vi "start cases.vi"() -> ()   [LabVIEW 2015]
panel:
  out "right pwm out":dbl
  out "left pwm out":dbl
  in  "Tab Control":T1(tab)
  in  "right 0":dbl
  in  "left 0":dbl
  in  "left 1":dbl
  in  "right 1":dbl
  in  "left 2 straight":dbl
  in  "right 2 straight":dbl
  in  "right 2 arc":dbl
  in  "left 2 arc":dbl
  in  "left 3 arc 1":dbl
  in  "right 3 arc 1":dbl
  in  "left 3 arc 2":dbl
  in  "right 3 arc 2":dbl
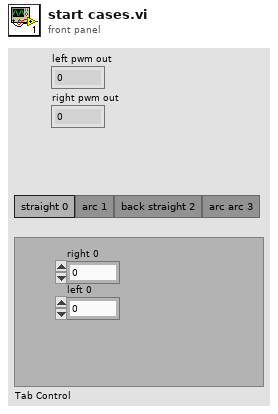
[diagram p1: front panel]
types:
  T1 = enum32{"straight 0", "arc 1", "back straight 2", "arc arc 3"}
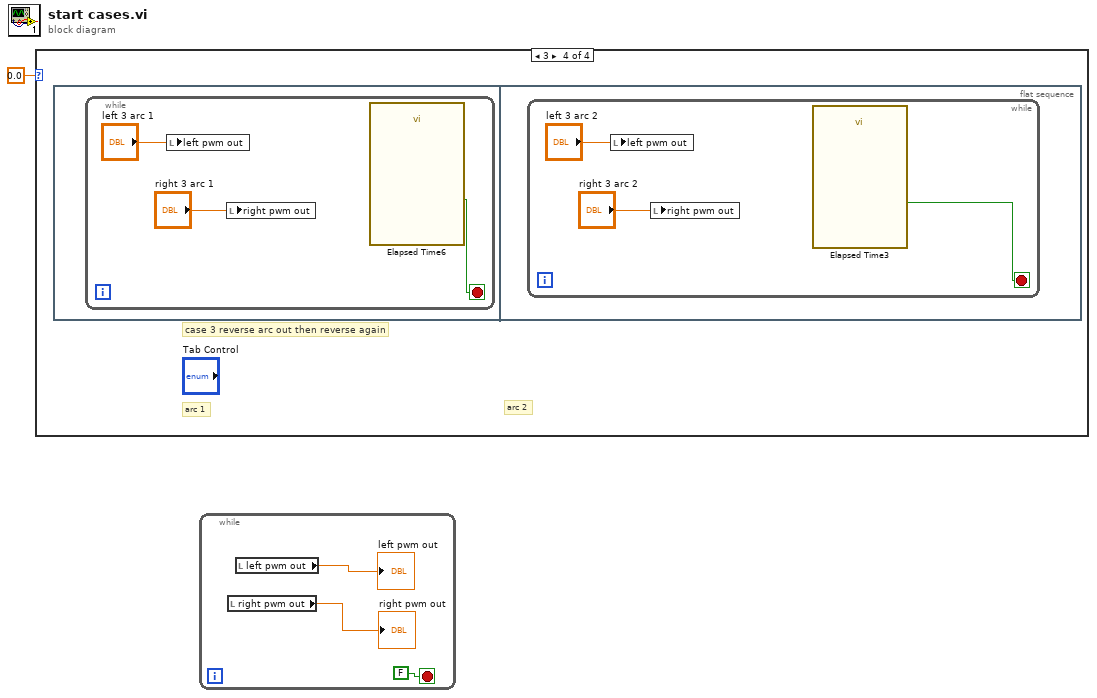
[diagram p0: block diagram]
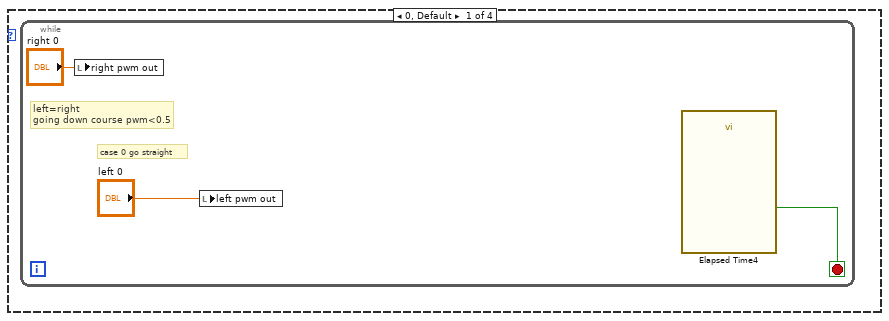
[diagram p2: hidden frame]
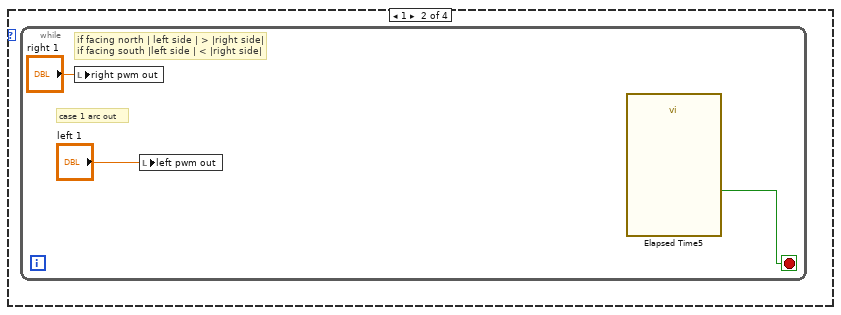
[diagram p3: hidden frame]
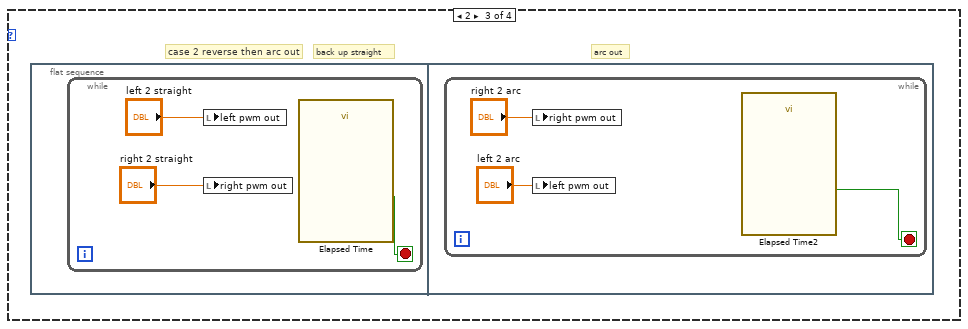
[diagram p4: hidden frame]
diagram:
  n1 = case shown="3" 0.0 {
    frame 0, Default {
      n2 = while {
        stop <- w2 stop-if-true
        # "left=right\ngoing down course pwm<0.5"
        # "case 0 go straight"
        n3 = local write "right pwm out"("right 0") -> ()
        n4 = local write "left pwm out"("left 0") -> ()
        n5 = call "Elapsed Time4"() -> ("Time has Elapsed"=w2:bool)  [unwired: 12 in, 7 out]
      }
    }
    frame 1 {
      n6 = while {
        stop <- w5 stop-if-true
        # "if facing north | left side | > |right side|\nif facing south |left side | < |right side|"
        # "case 1 arc out"
        n7 = local write "right pwm out"("right 1") -> ()
        n8 = local write "left pwm out"("left 1") -> ()
        n9 = call "Elapsed Time5"() -> ("Time has Elapsed"=w5:bool)  [unwired: 12 in, 7 out]
      }
    }
    frame 2 {
      # "arc out"
      # "back up straight"
      # "case 2 reverse then arc out"
      n10 = flat-sequence {
        frame #0 {
          n11 = while {
            stop <- w8 stop-if-true
            n12 = local write "left pwm out"("left 2 straight") -> ()
            n13 = local write "right pwm out"("right 2 straight") -> ()
            n14 = call "Elapsed Time"() -> ("Time has Elapsed"=w8:bool)  [unwired: 12 in, 7 out]
          }
        }
        frame #1 {
          n15 = while {
            stop <- w11 stop-if-true
            n16 = local write "right pwm out"("right 2 arc") -> ()
            n17 = local write "left pwm out"("left 2 arc") -> ()
            n18 = call "Elapsed Time2"() -> ("Time has Elapsed"=w11:bool)  [unwired: 12 in, 7 out]
          }
        }
      }
    }
    frame 3 {
      # "arc 2"
      # "arc 1"
      # "case 3 reverse arc out then reverse again"
      n19 = flat-sequence {
        frame #0 {
          n20 = while {
            stop <- w14 stop-if-true
            n21 = local write "left pwm out"("left 3 arc 1") -> ()
            n22 = local write "right pwm out"("right 3 arc 1") -> ()
            n23 = call "Elapsed Time6"() -> ("Time has Elapsed"=w14:bool)  [unwired: 12 in, 7 out]
          }
        }
        frame #1 {
          n24 = while {
            stop <- w17 stop-if-true
            n25 = local write "left pwm out"("left 3 arc 2") -> ()
            n26 = local write "right pwm out"("right 3 arc 2") -> ()
            n27 = call "Elapsed Time3"() -> ("Time has Elapsed"=w17:bool)  [unwired: 12 in, 7 out]
          }
        }
      }
    }
  }
  n28 = while {
    stop <- FALSE stop-if-true
    n29 = local read "right pwm out"() -> (→"right pwm out":dbl)
    n30 = local read "left pwm out"() -> (→"left pwm out":dbl)
  }
